vi "Handle Messages.vi"(8 "error in (no error)":errorcluster, 9 "Message Data":variant, 10 "Message":string, 11 "Application In":refnum<class "Application.lvclass">) -> (0 "error out":errorcluster, 3 "Application Out":refnum<class "Application.lvclass">)   [LabVIEW 2020, in "Application.lvclass"]
doc: "This is the main method handling incomming messages to the process. This method should be overridden to add functionality to the process or override functionality implemented by a parent. Any message not handled should be sent to the parent method using the default case. \nEach state should be atomic and states should not enqueue new messages from within this method. For cyclic iteration of an action, using a Helper Loop is recommended."
uses:
  Application.lvclass
  Process/Process.lvclass
  C:/Users/anton/Documents/GitHub/Triarc-Framework/source/Framework/Base/Base.lvclass
  C:/Users/anton/Documents/GitHub/Triarc-Framework/source/Framework/Process/Process.lvclass
  C:/Users/anton/Documents/GitHub/Triarc-Framework/source/Framework/Error Handler Interface/Error Handler Interface.lvclass
  C:/Users/anton/Documents/GitHub/Triarc-Framework/source/Framework/Logging/Logging.lvclass
  C:/Users/anton/Documents/GitHub/Triarc-Framework/source/Framework/Application/Application.lvclass
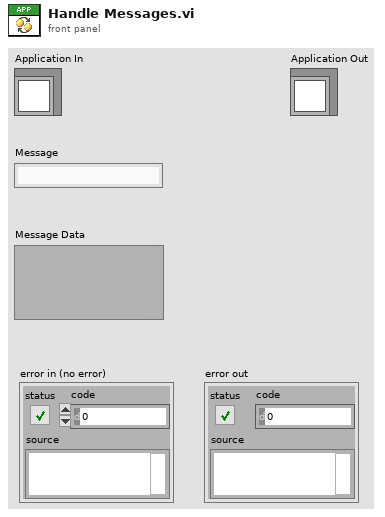
[diagram p1: front panel]
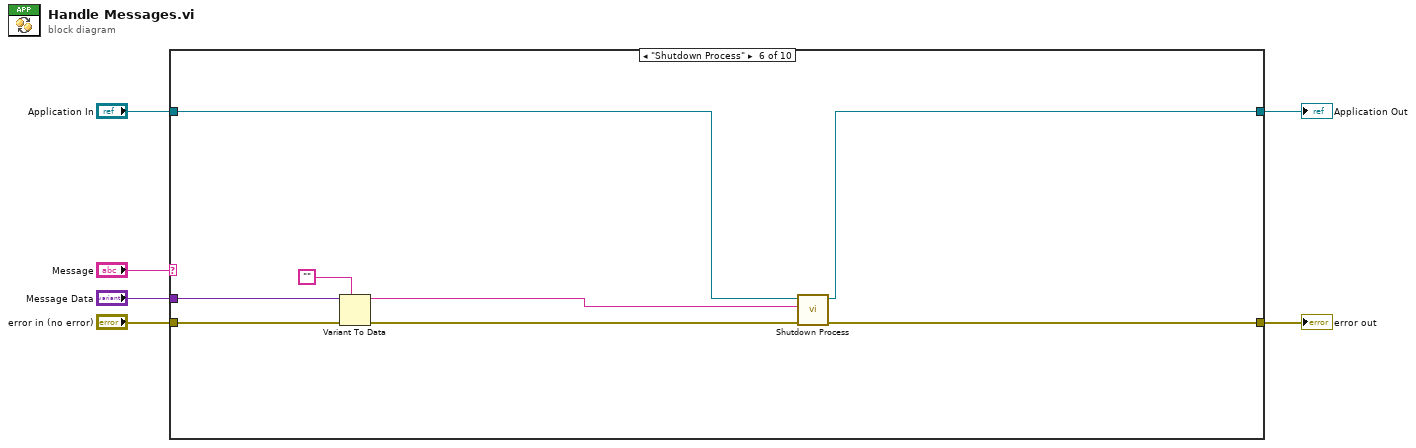
[diagram p0: block diagram]
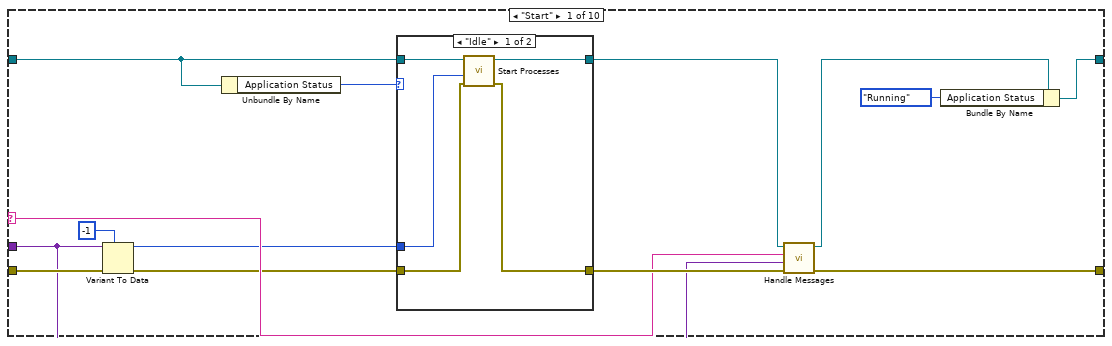
[diagram p2: hidden frame]
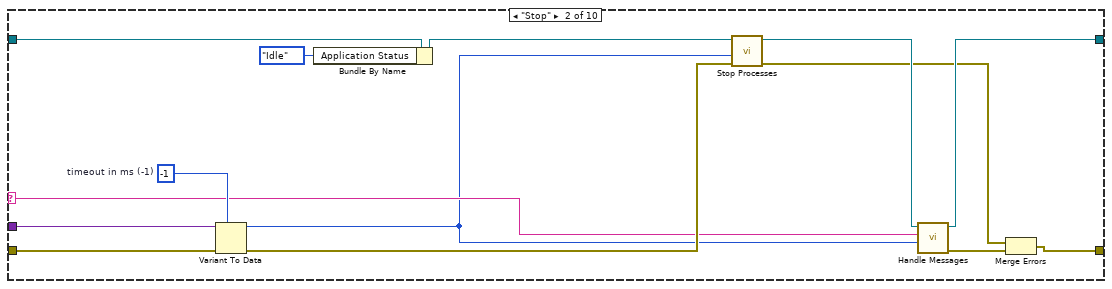
[diagram p4: hidden frame]
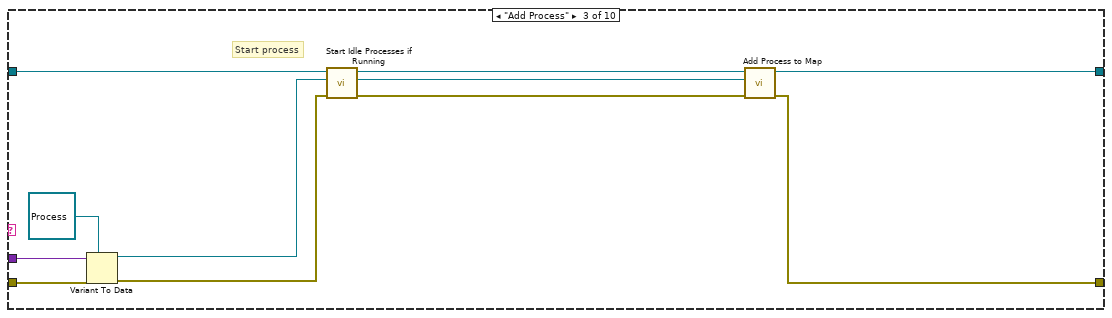
[diagram p5: hidden frame]
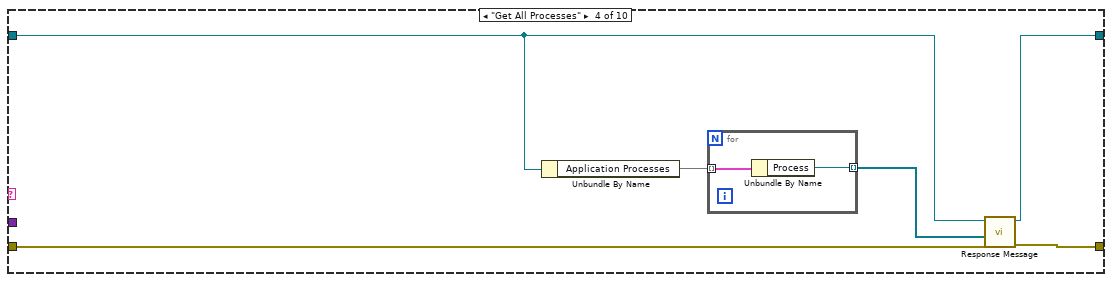
[diagram p6: hidden frame]
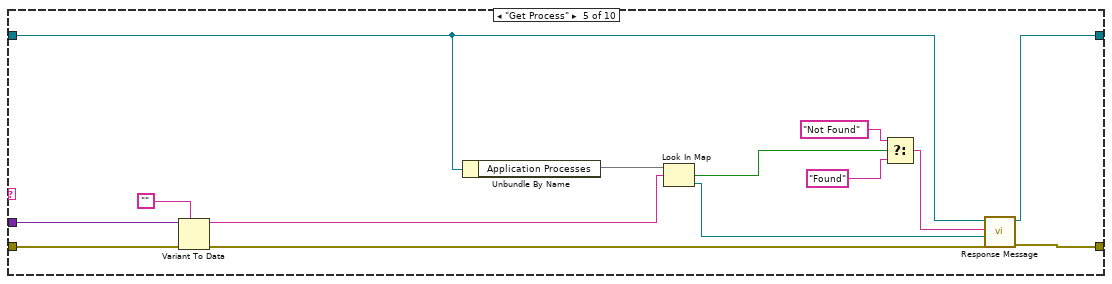
[diagram p7: hidden frame]
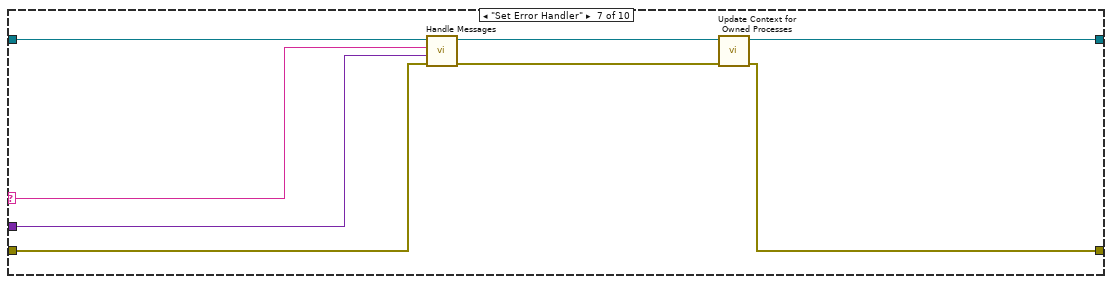
[diagram p8: hidden frame]
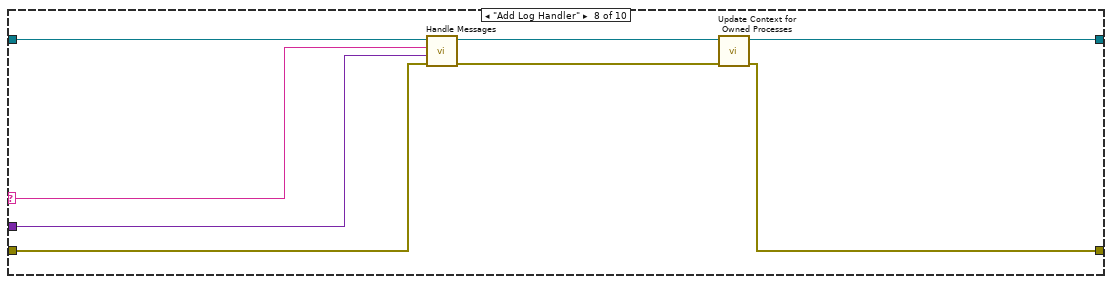
[diagram p9: hidden frame]
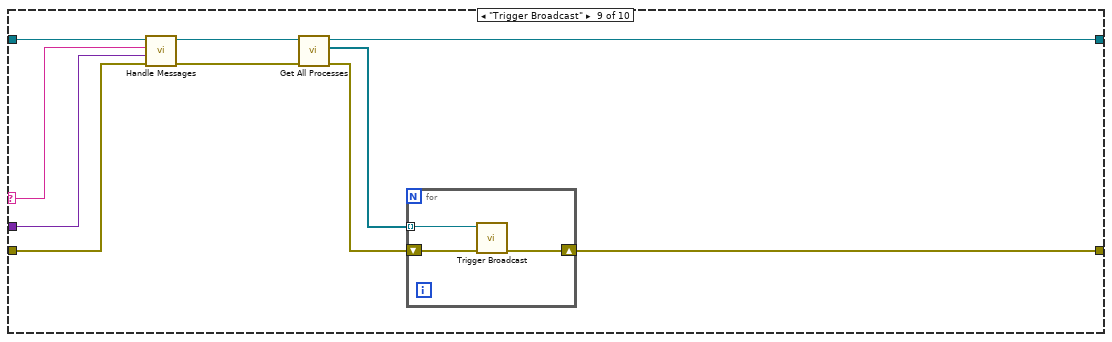
[diagram p10: hidden frame]
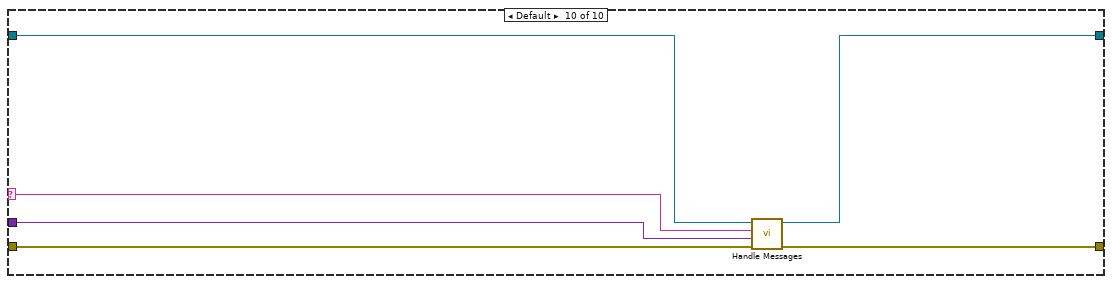
[diagram p11: hidden frame]
diagram:
  n1 = case shown="\"Shutdown Process\"" "Message" {
    selector: "Message" -> [w17 w33 _ _ _ _ w89 w97 w105 w113]
    tunnel: [w19 w28 w50 w56 w72 w78 w86 w94 w99 w117] -> w6
    tunnel: [w14 w34 w42 w55 w71 w75 w85 w93 w103 w116] -> w1
    tunnel: "error in (no error)" -> [w11 w41 w51 w58 w74 w82 w84 w92 w106 w115]
    tunnel: "Message Data" -> [w7 w40 w52 _ w68 w80 w88 w96 w104 w114]
    tunnel: "Application In" -> [w13 w37 w46 w54 w70 w77 w90 w98 w108 w112]
    frame "Start" {
      n2 = Variant To Data(error in=w11, type=-1 ("Timeout [ms] (-1)"), Variant=w7) -> (data=w8:i32, error out=w10:errorcluster)
      n3 = Unbundle By Name(w13) -> ("Application Status"=w12:enum16{"Idle", "Running"})
      n4 = case shown="\"Idle\"" w12 {
        tunnel: w10 -> [w25 w26]
        tunnel: [w24 w26] -> w20
        tunnel: [w23 w27] -> w18
        tunnel: w13 -> [w22 w27]
        tunnel: w8 -> [w21 _]
        frame "Idle" {
          n5 = call "Start Processes.vi"("error in (no error)"=w25, "Timeout [ms] (-1)"=w21, "Rig in"=w22) -> ("error out"=w24:errorcluster, "Rig out"=w23:refnum<class "Application.lvclass">)  [unwired: 7 in]
        }
        frame "Running" {
        }
      }
      n6 = call-parent "Handle Messages.vi"("error in (no error)"=w20, "Message Data"=w7, "Message"=w17, "Process In"=w18) -> ("error out"=w19:errorcluster, "Process Out"=w15:refnum<class "Application.lvclass">)  [unwired: 6 in]
      n7 = Bundle By Name(cluster=w15, "Application Status"=enum16{"Idle", "Running"}."Running") -> (w14:refnum<class "Application.lvclass">)
    }
    frame "Stop" {
      w39 = -1  # timeout in ms (-1)
      n8 = Variant To Data(error in=w41, type=w39, Variant=w40) -> (data=w32:i32, error out=w38:errorcluster)
      n9 = Bundle By Name(cluster=w37, "Application Status"=enum16{"Idle", "Running"}."Idle") -> (w30:refnum<class "Application.lvclass">)
      n10 = call "Stop Processes.vi"("error in (no error)"=w38, "timeout in ms (-1)"=w32, "Application In"=w30) -> ("error out"=w31:errorcluster, "Application Out"=w35:refnum<class "Application.lvclass">)  [unwired: 6 in, 1 out]
      n11 = call-parent "Handle Messages.vi"("Message Data"=w32, "Message"=w33, "Process In"=w35) -> ("error out"=w36:errorcluster, "Process Out"=w34:refnum<class "Application.lvclass">)  [unwired: 7 in]
      n12 = Merge Errors(w31, w36) -> (w28:errorcluster)
    }
    frame "Add Process" {
      # "Start process"
      n13 = Variant To Data(error in=w51, type=refnum<class "Process.lvclass"> refnum ("Rig Process"), Variant=w52) -> (data=w48:refnum<class "Process.lvclass">, error out=w47:errorcluster)
      n14 = call "Start Idle Processes if Running.vi"("error in (no error)"=w47, "Rig Process"=w48, "Rig in"=w46) -> ("error out"=w43:errorcluster, "Rig Process Out"=w45:refnum<class "Process.lvclass">, "Rig out"=w44:refnum<class "Application.lvclass">)  [unwired: 6 in]
      n15 = call "Add Process to Map.vi"("error in (no error)"=w43, "Process Out"=w45, "Application in"=w44) -> ("error out"=w50:errorcluster, "Application out"=w42:refnum<class "Application.lvclass">)  [unwired: 7 in]
    }
    frame "Get All Processes" {
      n16 = Unbundle By Name(w54) -> ("Application Processes"=w57:map{string, refnum<class "Process.lvclass">})
      n17 = for {
        tunnel: w57 -> [w60] mode=indexing
        tunnel: [w59] -> w53 mode=indexing
        n18 = Unbundle By Name(w60) -> ("Process"=w59:refnum<class "Process.lvclass">)
      }
      n19 = call "Response Message.vi"("error in (no error)"=w58, "Response Message Data"=w53, "Process In"=w54) -> ("error out"=w56:errorcluster, "Process Out"=w55:refnum<class "Application.lvclass">)  [unwired: 7 in]
    }
    frame "Get Process" {
      n20 = Variant To Data(error in=w74, type="", Variant=w68) -> (data=w66:string, error out=w69:errorcluster)
      n21 = Unbundle By Name(w70) -> ("Application Processes"=w73:map{string, refnum<class "Process.lvclass">})
      n22 = Look In Map(map=w73, key=w66) -> (key not found?=w62:bool, value=w65:refnum<class "Process.lvclass">)  [unwired: 1 in]
      n23 = Select(t="Not Found", s=w62, f="Found") -> (s? t:f=w61:string)
      n24 = call "Response Message.vi"("error in (no error)"=w69, "Response Message Data"=w65, "Response Message"=w61, "Process In"=w70) -> ("error out"=w72:errorcluster, "Process Out"=w71:refnum<class "Application.lvclass">)  [unwired: 6 in]
    }
    frame "Shutdown Process" {
      n25 = Variant To Data(error in=w82, type="", Variant=w80) -> (data=w76:string, error out=w81:errorcluster)
      n26 = call "Shutdown Process.vi"("error in (no error)"=w81, "Process Name"=w76, "Rig In"=w77) -> ("error out"=w78:errorcluster, "Rig Out"=w75:refnum<class "Application.lvclass">)  [unwired: 7 in]
    }
    frame "Set Error Handler" {
      n27 = call-parent "Handle Messages.vi"("error in (no error)"=w84, "Message Data"=w88, "Message"=w89, "Process In"=w90) -> ("error out"=w83:errorcluster, "Process Out"=w87:refnum<class "Application.lvclass">)  [unwired: 6 in]
      n28 = call "Update Context for Owned Processes.vi"("error in (no error)"=w83, "Application In"=w87) -> ("error out"=w86:errorcluster, "Application Out"=w85:refnum<class "Application.lvclass">)  [unwired: 8 in]
    }
    frame "Add Log Handler" {
      n29 = call-parent "Handle Messages.vi"("error in (no error)"=w92, "Message Data"=w96, "Message"=w97, "Process In"=w98) -> ("error out"=w91:errorcluster, "Process Out"=w95:refnum<class "Application.lvclass">)  [unwired: 6 in]
      n30 = call "Update Context for Owned Processes.vi"("error in (no error)"=w91, "Application In"=w95) -> ("error out"=w94:errorcluster, "Application Out"=w93:refnum<class "Application.lvclass">)  [unwired: 8 in]
    }
    frame "Trigger Broadcast" {
      n31 = call-parent "Handle Messages.vi"("error in (no error)"=w106, "Message Data"=w104, "Message"=w105, "Process In"=w108) -> ("error out"=w102:errorcluster, "Process Out"=w107:refnum<class "Application.lvclass">)  [unwired: 6 in]
      n32 = call "Get All Processes.vi"("error in (no error)"=w102, "Application In"=w107) -> ("error out"=w100:errorcluster, "App Processes"=w101:refnum<class "Process.lvclass">[], "Application Out"=w103:refnum<class "Application.lvclass">)  [unwired: 7 in]
      n33 = for {
        tunnel: w101 -> [w111] mode=indexing
        shift-right: [w109] -> w99
        shift-left: w100 -> [w110]
        n34 = call "Trigger Broadcast.vi"("error in (no error)"=w110, "Process in"=w111) -> ("error out"=w109:errorcluster)  [unwired: 8 in, 1 out]
      }
    }
    frame Default {
      n35 = call-parent "Handle Messages.vi"("error in (no error)"=w115, "Message Data"=w114, "Message"=w113, "Process In"=w112) -> ("error out"=w117:errorcluster, "Process Out"=w116:refnum<class "Application.lvclass">)  [unwired: 6 in]
    }
  }
  "error out" <- w6
  "Application Out" <- w1
